vi "Initialize.vi"(8 "error in (no error)":errorcluster, 10 "parent":string, 11 "file handler in":refnum<class "File Handler.lvclass">) -> (0 "error out":errorcluster, 2 "name":string, 3 "file handler out":refnum<class "File Handler.lvclass">)   [LabVIEW 2018, in "GLog.lvlib" / "File Handler.lvclass"]
uses:
  File Handler.lvclass
  File Handler.lvclass/File Handler.ctl
  extension/formatting_handler_interface/Formatting Handler.lvclass
panel:
  # "Connector Pane"
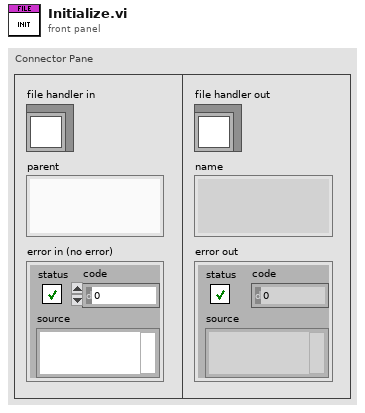
[diagram p1: front panel]
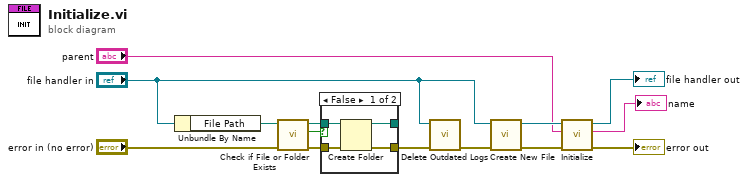
[diagram p0: block diagram]
diagram:
  n1 = Unbundle By Name("file handler in") -> ("File Path"=w12:path)
  n2 = call <vilib>:"Check if File or Folder Exists.vi"("error in (no error)"="error in (no error)", "path"=w12) -> ("error out"=w8:errorcluster, "file or folder exists?"=w7:bool, "dup path"=w6:path)  [unwired: 7 in]
  n3 = case shown="False" w7 {
    tunnel: [w16 w20] -> w11
    tunnel: w8 -> [w18 w20]
    tunnel: w6 -> [w17 w19]
    tunnel: [w15 w19] -> _
    frame False {
      n4 = Create Folder(path (use dialog)=w17, error in=w18) -> (created path=w15:path, error out=w16:errorcluster)  [unwired: 1 in, 1 out]
    }
    frame True {
    }
  }
  n5 = call "Delete Outdated Logs.vi"("error in (no error)"=w11, "file handler in"="file handler in") -> ("error out"=w10:errorcluster)  [unwired: 9 in]
  n6 = call "Create New File.vi"("error in (no error)"=w10, "file handler in"="file handler in") -> ("error out"=w14:errorcluster, "file handler out"=w4:refnum<class "File Handler.lvclass">)  [unwired: 8 in]
  n7 = call-parent "Initialize.vi"("error in (no error)"=w14, "parent"="parent", "handler in"=w4) -> ("error out"=→"error out":errorcluster, "name"=→"name":string, "handler out"=→"file handler out":refnum<class "File Handler.lvclass">)  [unwired: 6 in]
